vi "OAT Auto Spectrogram Range.vi"(6 "type":T1(ring)=enum."Order-RPM", 8 "error in (no error)":errorcluster, 10 "speed profile in":T3 {"speed [RPM]" format="%.2f"; "time [s]" format="%.2f"}, 11 "scaled signal [EU] in":waveform(dbl)) -> (0 "error out":errorcluster, 2 "speed profile out":T3 {"speed [RPM]" format="%.2f"; "time [s]" format="%.2f"}, 3 "scaled signal [EU] out":waveform(dbl), 4 "config":T2={"type"=enum."Order-RPM", "range"={"start"=0.0, "end"=0.0, "step"=0.0}} {"range"."step" format="%.2f"; "range"."end" format="%.2f"; "range"."start" format="%.2f"})   [LabVIEW 2017]
uses:
  <vilib>/addons/Sound and Vibration/Order Analysis/Tach Process/SubVIs/speed profile.ctl
  <vilib>/addons/Sound and Vibration/Order Analysis/Tach Process/SoundVib_TachProcess.lvlib
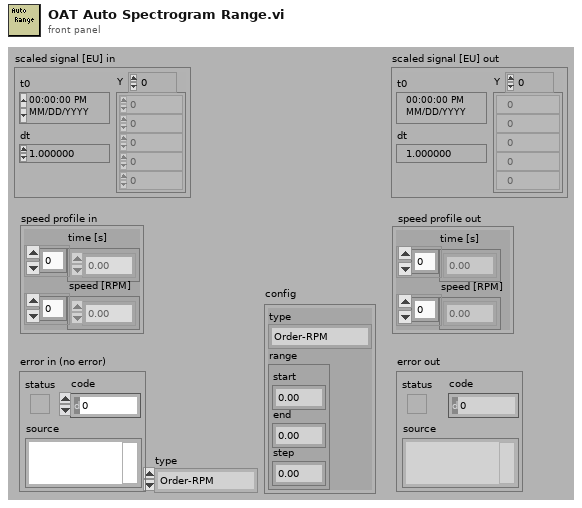
[diagram p1: front panel]
types:
  T1 = enum16{"Frequency-Time", "Frequency-RPM", "Order-RPM"}
  T2 = cluster{"type":enum16{"Frequency-Time", "Frequency-RPM", "Order-RPM"}, "range":cluster{"start":dbl, "end":dbl, "step":dbl}}
  T3 = typedef "SoundVib_TachProcess.lvlib/speed profile.ctl" = cluster{"time [s]":dbl[], "speed [RPM]":dbl[]}
  T4 = cluster{"Minimum":dbl, "Maximum":dbl, "Increment":dbl}
  T5 = cluster{"type":enum16{"Frequency-Time", "Frequency-RPM", "Order-RPM"}, "RPM range out":cluster{"Minimum":dbl, "Maximum":dbl, "Increment":dbl}}
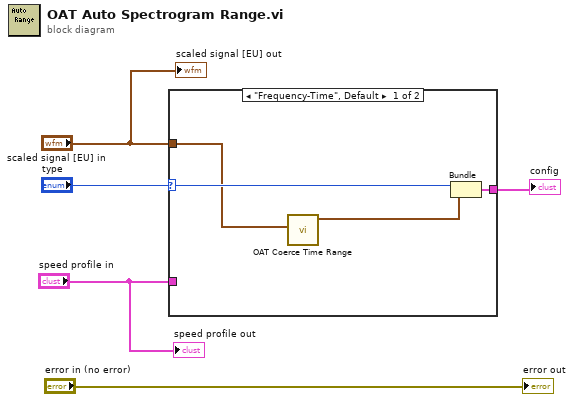
[diagram p0: block diagram]
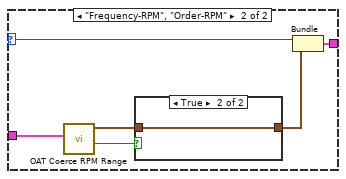
[diagram p2: hidden frame]
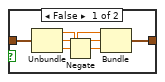
[diagram p3: hidden frame]
diagram:
  n1 = case shown="\"Frequency-Time\", Default" "type" {
    selector: "type" -> [w9 w13]
    tunnel: "speed profile in" -> [_ w10]
    tunnel: [w6 w12] -> w4
    tunnel: "scaled signal [EU] in" -> [w8 _]
    frame "Frequency-Time", Default {
      n2 = call <vilib>:"OAT Coerce Time Range.vi"("scaled signal [EU] in"=w8) -> ("RPM range out"=w7:T4)  [unwired: 5 in, 1 out]
      n3 = Bundle("type"=w9, "RPM range out"=w7) -> (w6:T5)  [unwired: 1 in]
    }
    frame "Frequency-RPM", "Order-RPM" {
      n4 = call <vilib>:"OAT Coerce RPM Range.vi"("speed profile"=w10) -> ("run up?"=w15:bool, "RPM range out"=w11:T4)  [unwired: 4 in, 1 out]
      n5 = case shown="True" w15 {
        tunnel: w11 -> [w17 w22]
        tunnel: [w16 w22] -> w14
        frame False {
          n6 = Unbundle(w17) -> ("Minimum"=w21:dbl, "Maximum"=w20:dbl, "Increment"=w19:dbl)
          n7 = Negate(x=w19) -> (-x=w18:dbl)
          n8 = Bundle(cluster=w17, "Minimum"=w20, "Maximum"=w21, "Increment"=w18) -> (w16:T4)
        }
        frame True {
        }
      }
      n9 = Bundle("type"=w13, "RPM range out"=w14) -> (w12:T5)  [unwired: 1 in]
    }
  }
  "config" <- w4
  "scaled signal [EU] out" <- "scaled signal [EU] in"
  "speed profile out" <- "speed profile in"
  "error out" <- "error in (no error)"
